vi "Example Monitor.vi"() -> ()   [LabVIEW 2020, in "Jasco UV.lvlib"]
uses:
  Jasco UV.lvlib
panel:
  out "String out":string
  in  "Stop":bool
  in  "VISA resource\n name":refnum<visa-resource-name>
  out "Waveform Chart":ext(graph)
  in  "Integrator Output\n Range":T1(ring)
  in  "Auto Zero Pos":enum16{"0", "5", "10", "50", "100"}(ring)
  in  "Auto Zero":enum16{"AUTO", "MANUAL", "HOLD"}(ring)
  in  "Response":enum16{"FAST", "STD", "SLOW"}(ring)
  in  "Range":T2(ring)
  in  "Signal Filter":enum16{"Time Acc", "CR", "Digital"}(ring)
  in  "Polarity":enum16{"Plus", "Minus"}(ring)
  in  "Wavelength (nm)":u32=190 min=190 max=600 step=1
  in  "Program File No.":u32 max=9 step=1
  out "Absorbance (ABU)":dbl
  in  "Sampling Time (ms)":u32=250
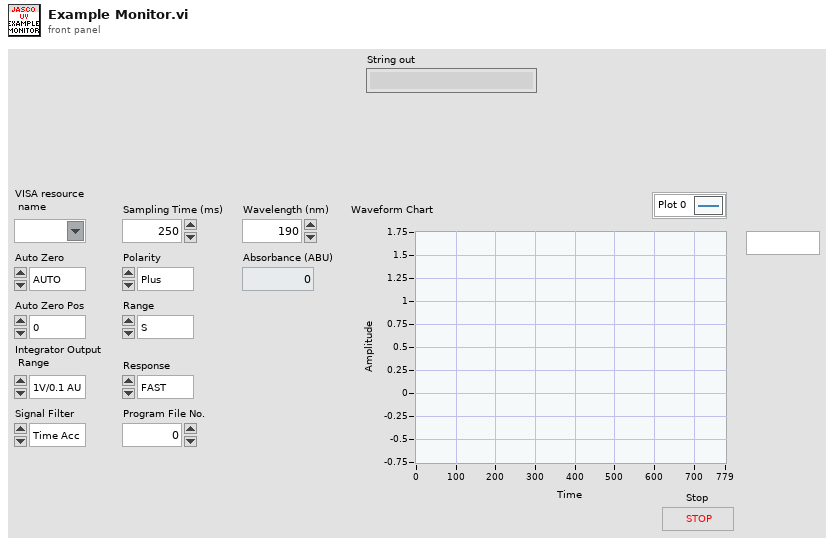
[diagram p1: front panel]
types:
  T1 = enum16{"1V/0.1 AU", "1V/1.0 AU", "1V/2.0 AU", "1V/3.0 AU"}
  T2 = enum16{"S", "2.56", "1.28", "0.64", "0.32", "0.16", "0.08", "0.04", "0.02", "0.01", "0.005", "0.0025", "0.00125", "0.0005"}
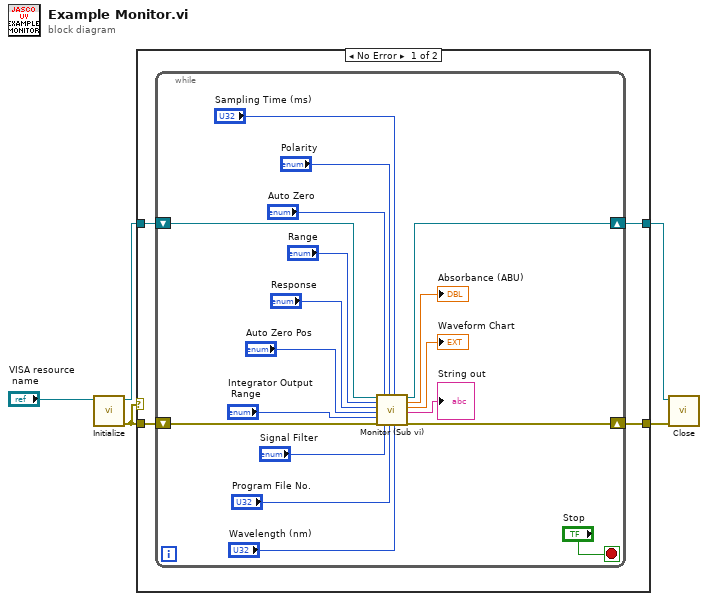
[diagram p0: block diagram]
diagram:
  n1 = call "Initialize.vi"("VISA resource name"="VISA resource\n name") -> ("error out"=w1:errorcluster, "VISA resource name out"=w4:refnum<visa-resource-name>)  [unwired: 9 in]
  n2 = case shown="No Error" w1 {
    tunnel: w1 -> [w9 w28]
    tunnel: w4 -> [w8 w29]
    tunnel: [w7 w29] -> w3
    tunnel: [w6 w28] -> w2
    frame No Error {
      n3 = while {
        shift-right: [w14] -> w7
        shift-left: w8 -> [w26]
        shift-right: [w13] -> w6
        shift-left: w9 -> [w25]
        stop <- "Stop" stop-if-true
        n4 = call "Monitor (Sub vi).vi"("VISA Refnum in"=w26, "Range"="Range", "Response"="Response", "Auto Zero Pos"="Auto Zero Pos", "Integrator Output\n Range"="Integrator Output\n Range", "error in (no error)"=w25, "Auto Zero"="Auto Zero", "Signal Filter"="Signal Filter", "Polarity"="Polarity", "Program File No."="Program File No.", "Sampling Time (ms)"="Sampling Time (ms)", "Wavelength (nm)"="Wavelength (nm)") -> ("VISA Refnum out"=w14:refnum<visa-resource-name>, "Absorbance (ABU)"=→"Absorbance (ABU)":dbl, "Waveform Chart"=→"Waveform Chart":ext, "String out"=→"String out":string, "error out"=w13:errorcluster)  [unwired: 3 in]
      }
    }
    frame Error {
    }
  }
  n5 = call "Close.vi"("error in (no error)"=w2, "VISA resource name"=w3) -> ()  [unwired: 9 in, 1 out]
